vi "Revision Query.vi"(8 "error in (no error)":errorcluster, 11 "VISA resource name":refnum<visa-resource-name>) -> (0 "error out":errorcluster, 1 "Instrument Firmware Revision":string, 2 "Instrument Driver Revision":string, 3 "VISA resource name out":refnum<visa-resource-name>)   [LabVIEW 2014, in "GRBLMotionCore.lvlib"]
doc: "Queries the current instrument firmware revision and instrument driver revision.\n\nRefer to the Readme file for detailed driver information including modification history."
uses:
  <instrlib>/GRBL/GRBLMotionCore.lvlib
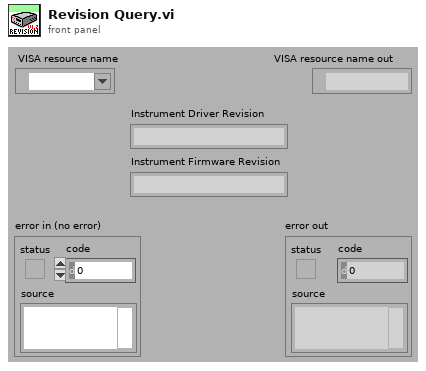
[diagram p1: front panel]
types:
  T1 = enum32{"invalid app kind", "Development System", "Run Time System", "Student Edition", "Embedded LabVIEW", "Evaluation", "Custom"}
  T2 = cluster{"Major":u16, "Minor":u16, "Fix":u16, "Build":u16}
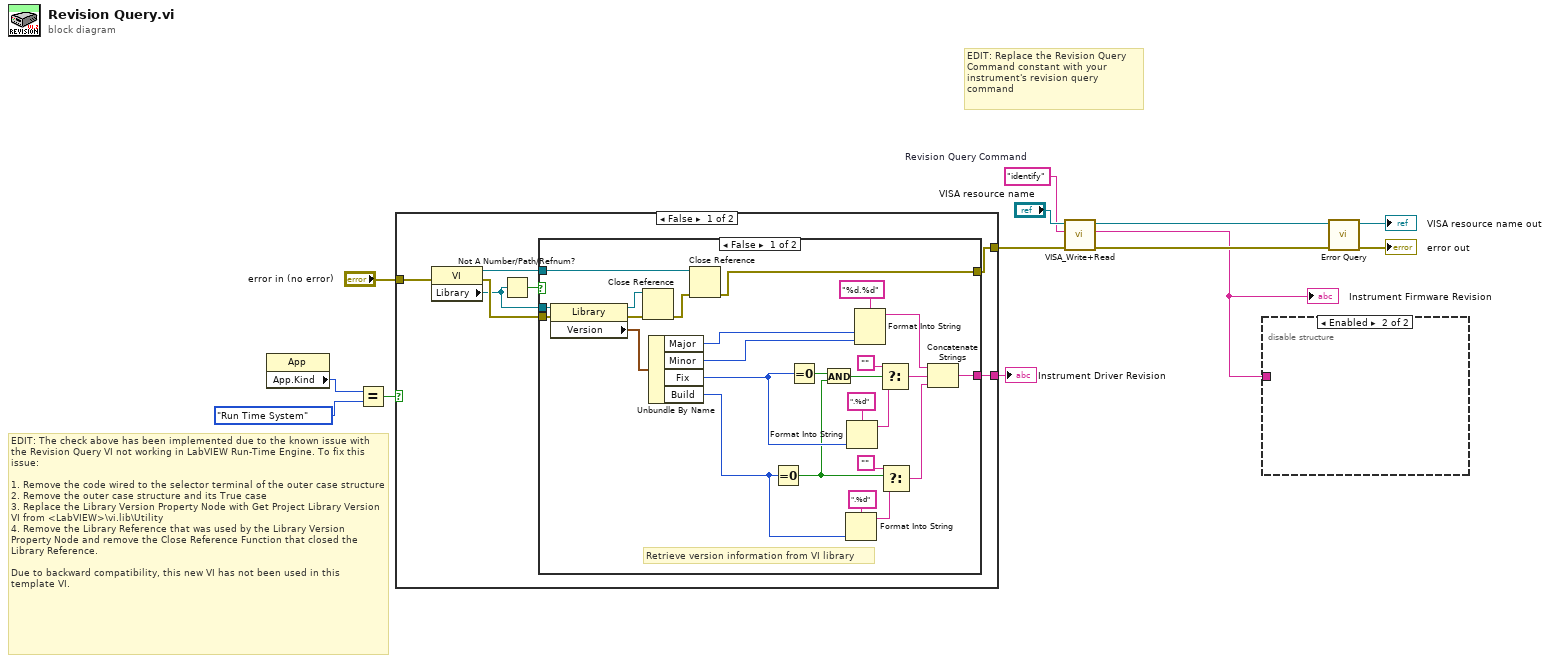
[diagram p0: block diagram]
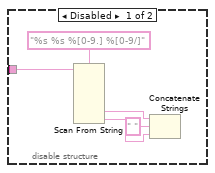
[diagram p2: hidden frame]
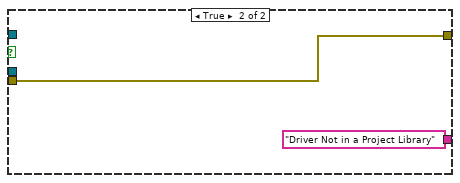
[diagram p3: hidden frame]
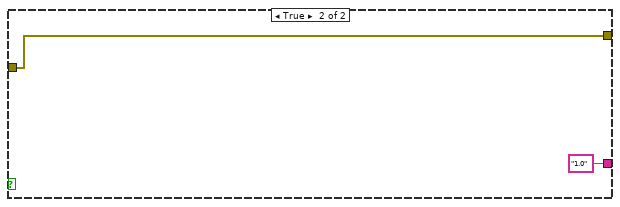
[diagram p4: hidden frame]
diagram:
  w10 = "identify"  # Revision Query Command
  # "EDIT: The check above has been implemented due to the known issue with the Revision Query VI not working in LabVIEW Run-Time Engine. To fix this issue:\n\n1. Remove the code wired to the selector terminal of the outer case structure\n2. Remove the outer case structure and its True case\n3. Replace the Library Version Property Node with Get Project Library Version VI from <LabVIEW>\\vi.lib\\Utility\n4. Remove the Library Reference that was used by the Library Version Property Node and remove the Close Reference Function that closed the Library Reference.\n\nDue to backward compatibility, this new VI has not been used in this template VI."
  # "EDIT: Replace the Revision Query\nCommand constant with your\ninstrument's revision query\ncommand"
  n1 = property class="App"() -> ("App.Kind"=w3:T1)  [unwired: 2 in, 2 out]
  n2 = Equal?(x=w3, y=T1."Run Time System" ("Application:Kind")) -> (x = y?=w4:bool)
  n3 = case shown="False" w4 {
    tunnel: [w16 "1.0"] -> w7
    tunnel: "error in (no error)" -> [w15 w49]
    tunnel: [w14 w49] -> w5
    frame False {
      n4 = property class="VI"(error in=w15) -> (reference out=w20:refnum<vi>, error out=w19:errorcluster, "Library"=w18:refnum<vi>)  [unwired: 1 in]
      n5 = Not A Number/Path/Refnum?(number/path/refnum=w18) -> (NaN/Path/Refnum?=w17:bool)
      n6 = case shown="False" w17 {
        tunnel: w20 -> [w43 _]
        tunnel: w19 -> [w28 w48]
        tunnel: [w23 w48] -> w14
        tunnel: [w22 "Driver Not in a Project Library"] -> w16
        tunnel: w18 -> [w21 _]
        frame False {
          # "Retrieve version information from VI library"
          n7 = property class="Library"(reference=w21, error in=w28) -> (reference out=w45:refnum<vi>, error out=w46:errorcluster, "Version"=w42:T2)
          n8 = Close Reference(reference=w45, error in (no error)=w46) -> (error out=w44:errorcluster)
          n9 = Unbundle By Name(w42) -> ("Major"=w31:u16, "Minor"=w30:u16, "Fix"=w27:u16, "Build"=w29:u16)
          n10 = Close Reference(reference=w43, error in (no error)=w44) -> (error out=w23:errorcluster)
          n11 = Equal To 0?(x=w29) -> (x = 0?=w25:bool)
          n12 = Equal To 0?(x=w27) -> (x = 0?=w26:bool)
          n13 = And(x=w26, y=w25) -> (x .and. y?=w24:bool)
          n14 = Format Into String(format string=".%d", w29) -> (resulting string=w35:string)  [unwired: 2 in, 1 out]
          n15 = Format Into String(format string=".%d", w27) -> (resulting string=w39:string)  [unwired: 2 in, 1 out]
          n16 = Format Into String(format string="%d.%d", w31, w30) -> (resulting string=w37:string)  [unwired: 2 in, 1 out]
          n17 = Select(t="", s=w24, f=w39) -> (s? t:f=w36:string)
          n18 = Select(t="", s=w25, f=w35) -> (s? t:f=w32:string)
          n19 = Concatenate Strings(w37, w36, w32) -> (w22:string)
        }
        frame True {
        }
      }
    }
    frame True {
    }
  }
  "Instrument Driver Revision" <- w7
  n20 = call <instrlib>:"VISA_Write+Read.vi"("error in (no error)"=w5, "Write Buffer"=w10, "VISA resource name"="VISA resource name") -> ("error out"=w11:errorcluster, "readout"=w1:string, "VISA resource name out"=w12:refnum<visa-resource-name>)  [unwired: 6 in]
  "Instrument Firmware Revision" <- w1
  n21 = disable-structure shown="Enabled" {
    disable-tunnel: w1 -> [w51 _]
    frame Disabled {
      n22 = Scan From String(format string="%s %s %[0-9.] %[0-9/]", input string=w51) -> (output 3=w54:string, output 4=w53:string)  [unwired: 8 in, 3 out]
      n23 = Concatenate Strings(w54, " " ("string"), w53) -> ()  [unwired: 1 out]
    }
    frame Enabled {
    }
  }
  n24 = call <instrlib>:"Error Query.vi"("error in (no error)"=w11, "VISA resource name"=w12) -> ("error out"=→"error out":errorcluster, "VISA resource name out"=→"VISA resource name out":refnum<visa-resource-name>)  [unwired: 6 in, 2 out]
